vi "sub_SDR_tx_ApplyShappingFilter.vi"(7 "Filter Options":T1={"Samples per symbol"=2, "Roll-Off"=1.0, "Filter length (symbols)"=4}, 10 "Data Symbols":cdb[](array[numeric])) -> (2 "Shaped symbols":cdb[](array[numeric]))   [LabVIEW 2012]
uses:
  <vilib>/Analysis/2dsp.llb/Upsample (CDB).vi
  <vilib>/Analysis/2dsp.llb/1D Convolution (CDB).vi
  <vilib>/Analysis/NI_AALPro.lvlib
  <vilib>/addons/Modulation/niDMT.lvlib
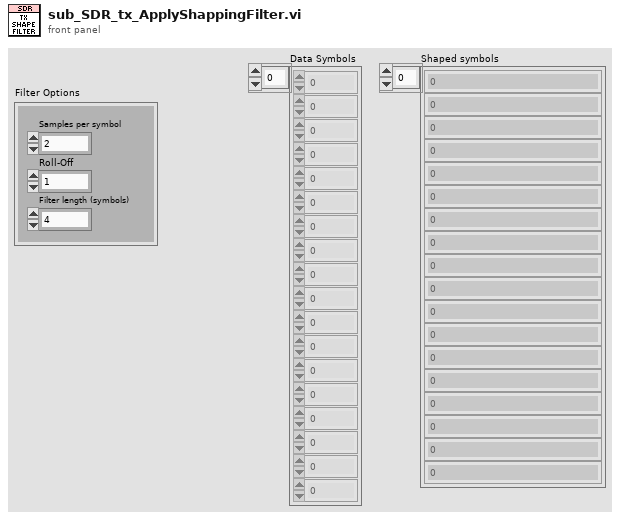
[diagram p1: front panel]
types:
  T1 = cluster{"Samples per symbol":i32, "Roll-Off":dbl, "Filter length (symbols)":i32}
  T2 = enum16{"FSK", "PSK", "QAM", "MSK", "PAM", "ASK", "CPM"}
  T3 = enum16{"none", "Raised Cosine", "Root Raised Cos", "Gaussian"}
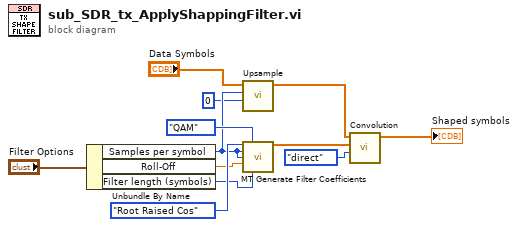
[diagram p0: block diagram]
diagram:
  n1 = Unbundle By Name("Filter Options") -> ("Samples per symbol"=w4:i32, "Roll-Off"=w7:dbl, "Filter length (symbols)"=w6:i32)
  n2 = call-poly <vilib>:"Upsample.vi"("leading zeros"=0, "upsampling factor"=w4, "X"="Data Symbols") -> ("Upsampled Array"=w2:cdb[])  [unwired: 7 in, 1 out]
  n3 = call <vilib>:"MT Generate Filter Coefficients.vi"("pulse shaping filter (none)"=T3."Root Raised Cos", "modulation type"=T2."QAM", "pulse shaping samples per symbol (16)"=w4, "matched samples per symbol (16)"=w4, "filter parameter"=w7, "filter length (symbols)"=w6) -> ("pulse shaping filter coefficients"=w5:dbl[])  [unwired: 7 in, 2 out]
  n4 = call-poly <vilib>:"Convolution.vi"("algorithm"=enum32{"direct", "frequency domain"}."direct", "Y"=w5, "X"=w2) -> ("X * Y"=→"Shaped symbols":cdb[])  [unwired: 7 in, 1 out]
